vi "1B Spoof Position Update.vi"(2 "dt":dbl, 3 "Simulator Bounds":T3={"Simulator E Range"=20.0, "Simulator E Min"=-10.0, "Simulator N Range"=20.0, "Simulator N Min"=-10.0}, 4 "Robot UTM Location":T1 {"North" format="%#_10f"; "East" format="%#_8f"}, 5 "Robot Velocity":T2) -> (0 "New Position (X,Y)":cluster{"X Position":dbl, "Y Position":dbl}, 1 "New Robot UTM Location":T1 {"North" format="%#_10f"; "East" format="%#_8f"})   [LabVIEW 2011]
uses:
  1,3 B Typedefs/simulator bounds.ctl
  2-Think/2 Typedefs/robot velocity.ctl
  2-Think/2 Typedefs/UTM Location.ctl
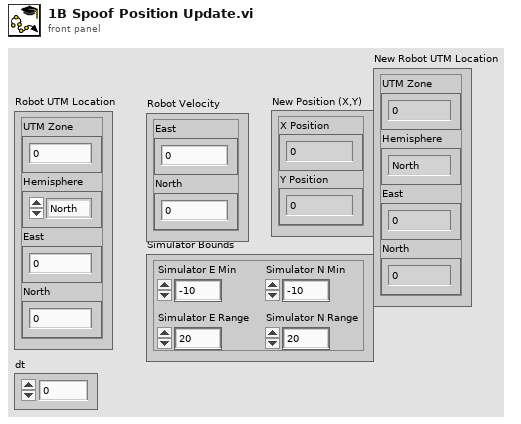
[diagram p1: front panel]
types:
  T1 = typedef "UTM Location.ctl" = cluster{"UTM Zone":dbl, "Hemisphere":enum16{"North", "South"}, "East":dbl, "North":dbl}
  T2 = typedef "robot velocity.ctl" = cluster{"East":dbl, "North":dbl}
  T3 = typedef "simulator bounds.ctl" = cluster{"Simulator E Range":dbl, "Simulator E Min":dbl, "Simulator N Range":dbl, "Simulator N Min":dbl}
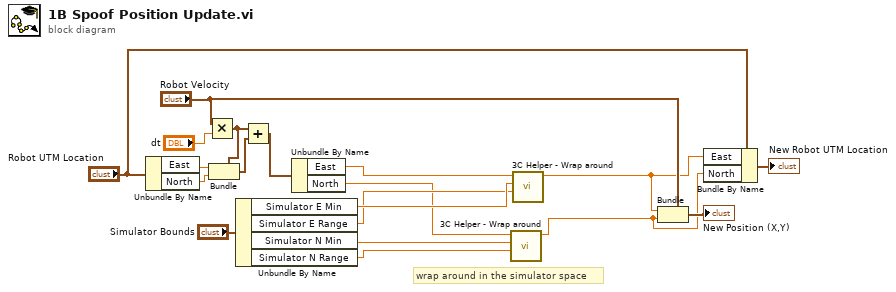
[diagram p0: block diagram]
diagram:
  # "wrap around in the simulator space"
  n1 = Unbundle By Name("Robot UTM Location") -> ("East"=w8:dbl, "North"=w7:dbl)
  n2 = Multiply(x="Robot Velocity", y="dt") -> (x*y=w5:T2)
  n3 = Bundle(cluster=w5, "East"=w8, "North"=w7) -> (w6:T2)
  n4 = Unbundle By Name("Simulator Bounds") -> ("Simulator E Min"=w16:dbl, "Simulator E Range"=w14:dbl, "Simulator N Min"=w11:dbl, "Simulator N Range"=w12:dbl)
  n5 = Add(x=w5, y=w6) -> (x+y=w17:T2)
  n6 = Unbundle By Name(w17) -> ("East"=w13:dbl, "North"=w10:dbl)
  n7 = call "3C Helper - Wrap around.vi"("Range allowed"=w12, "Min allowed"=w11, "Position in"=w10) -> ("Wrapped Position out"=w1:dbl)  [unwired: 8 in]
  n8 = call "3C Helper - Wrap around.vi"("Range allowed"=w14, "Min allowed"=w16, "Position in"=w13) -> ("Wrapped Position out"=w2:dbl)  [unwired: 8 in]
  n9 = Bundle(cluster="Robot Velocity", "East"=w2, "North"=w1) -> (→"New Position (X,Y)":T2)
  n10 = Bundle By Name(cluster="Robot UTM Location", "East"=w2, "North"=w1) -> (→"New Robot UTM Location":T1)
